vi "TCP Receive Packet.vi"(8 "error in (no error)":errorcluster, 10 "Packet Type":refnum<class "TCPPacket.lvclass">, 11 "TCP Refnum In":refnum<k5>) -> (0 "error out":errorcluster, 2 "TCPPacket":refnum<class "TCPPacket.lvclass">, 3 "TCP Refnum Out":refnum<k5>)   [LabVIEW 2019]
uses:
  TCPPacket/TCPPacket.lvclass
  TCPReceiver/TCPReceiver.lvclass
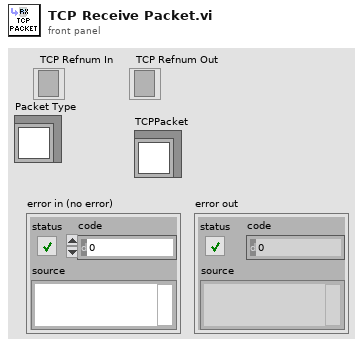
[diagram p1: front panel]
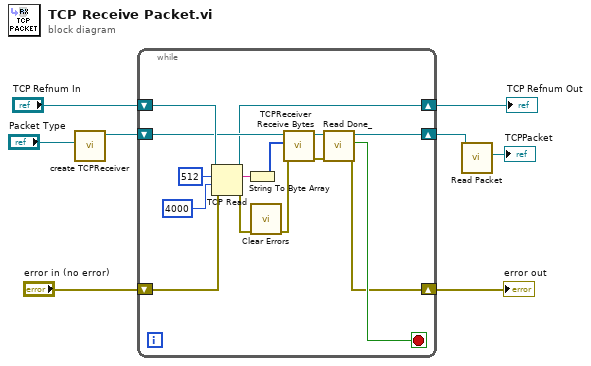
[diagram p0: block diagram]
diagram:
  n1 = call "create TCPReceiver.vi"("Packet Type"="Packet Type") -> ("TCPReceiver out"=w7:refnum<class "TCPReceiver.lvclass">)  [unwired: 9 in, 1 out]
  n2 = while {
    shift-right: [w12] -> w3
    shift-left: "TCP Refnum In" -> [w23]
    shift-right: [w13] -> w5
    shift-left: w7 -> [w19]
    shift-right: [w14] -> w2
    shift-left: "error in (no error)" -> [w21]
    stop <- w15 stop-if-true
    n3 = TCP Read(connection ID=w23, bytes to read=512, error in (no error)=w21, 9:4000 ("timeout ms (25000)")) -> (connection ID out=w12:refnum<k5>, data out=w20:string, error out=w10:errorcluster)  [unwired: 1 in]
    n4 = String To Byte Array(string=w20) -> (unsigned byte array=w18:u8[])
    n5 = call <vilib>:"Clear Errors.vi"("error in (no error)"=w10) -> ("error out"=w9:errorcluster)  [unwired: 5 in, 1 out]
    n6 = call-dynamic "TCPReceiver Receive Bytes.vi"("error in (no error)"=w9, "Data"=w18, "TCPReceiver in"=w19) -> ("error out"=w16:errorcluster, "TCPReceiver out"=w17:refnum<class "TCPReceiver.lvclass">)  [unwired: 7 in]
    n7 = call-dynamic "Read Done_.vi"("error in (no error)"=w16, "TCPReceiver in"=w17) -> ("error out"=w14:errorcluster, "Done?"=w15:bool, "TCPReceiver out"=w13:refnum<class "TCPReceiver.lvclass">)  [unwired: 7 in]
  }
  "TCP Refnum Out" <- w3
  "error out" <- w2
  n8 = call-dynamic "Read Packet.vi"("TCPReceiver in"=w5) -> ("TCPPacket.lvclass"=→"TCPPacket":refnum<class "TCPPacket.lvclass">)  [unwired: 8 in, 2 out]
